vi "test-trapezoid-profile-top-speed.vi"() -> ()   [LabVIEW 2019]
uses:
  <vilib>/Rock Robotics/WPI/ThirdParty/JAS_Junk/TrajLib/TRAPEZOID_PROFILE_STATE.ctl
  <vilib>/Rock Robotics/WPI/ThirdParty/JAS_Junk/TrajLib/TRAPEZOID_PROFILE.ctl
  <vilib>/Rock Robotics/WPI/ThirdParty/JAS_Junk/TrajLib/TRAPEZOID_PROFILE_CONSTRAINT.ctl
  <vilib>/Rock Robotics/WPI/ThirdParty/JAS_Junk/TrajLib/TrapProfile_ShouldFlipAcceleration.vi
  <vilib>/Rock Robotics/WPI/ThirdParty/JAS_Junk/TrajLib/TrapProfile_Direct.vi
  <vilib>/Rock Robotics/WPI/ThirdParty/JAS_Junk/TrajLib/Trajectory_Library.lvlib
panel:
  out "State 2":T1 {"Velocity" format="%16_6e"; "Position" format="%16_6e"}
  out "Waveform Chart 2":T2(graph)
  out "TRAPEZOID_PROFILE 2":T3 {"Goal"."Velocity" format="%16_6e"; "Goal"."Position" format="%16_6e"; "Initial"."Velocity" format="%16_6e"; "Initial"."Position" format="%16_6e"; "Constraints"."MaxAcceleration" format="%16_6e"; "Constraints"."MaxVelocity" format="%16_6e"; "EndDecel" format="%16_6e"; "EndFullSpeed" format="%16_6e"; "EndAccel" format="%16_6e"}
  out "TRAPEZOID_PROFILE":T3 {"Goal"."Velocity" format="%16_6e"; "Goal"."Position" format="%16_6e"; "Initial"."Velocity" format="%16_6e"; "Initial"."Position" format="%16_6e"; "Constraints"."MaxAcceleration" format="%16_6e"; "Constraints"."MaxVelocity" format="%16_6e"; "EndDecel" format="%16_6e"; "EndFullSpeed" format="%16_6e"; "EndAccel" format="%16_6e"}
  out "State":T1 {"Velocity" format="%16_6e"; "Position" format="%16_6e"}
  out "Waveform Chart":T2(graph)
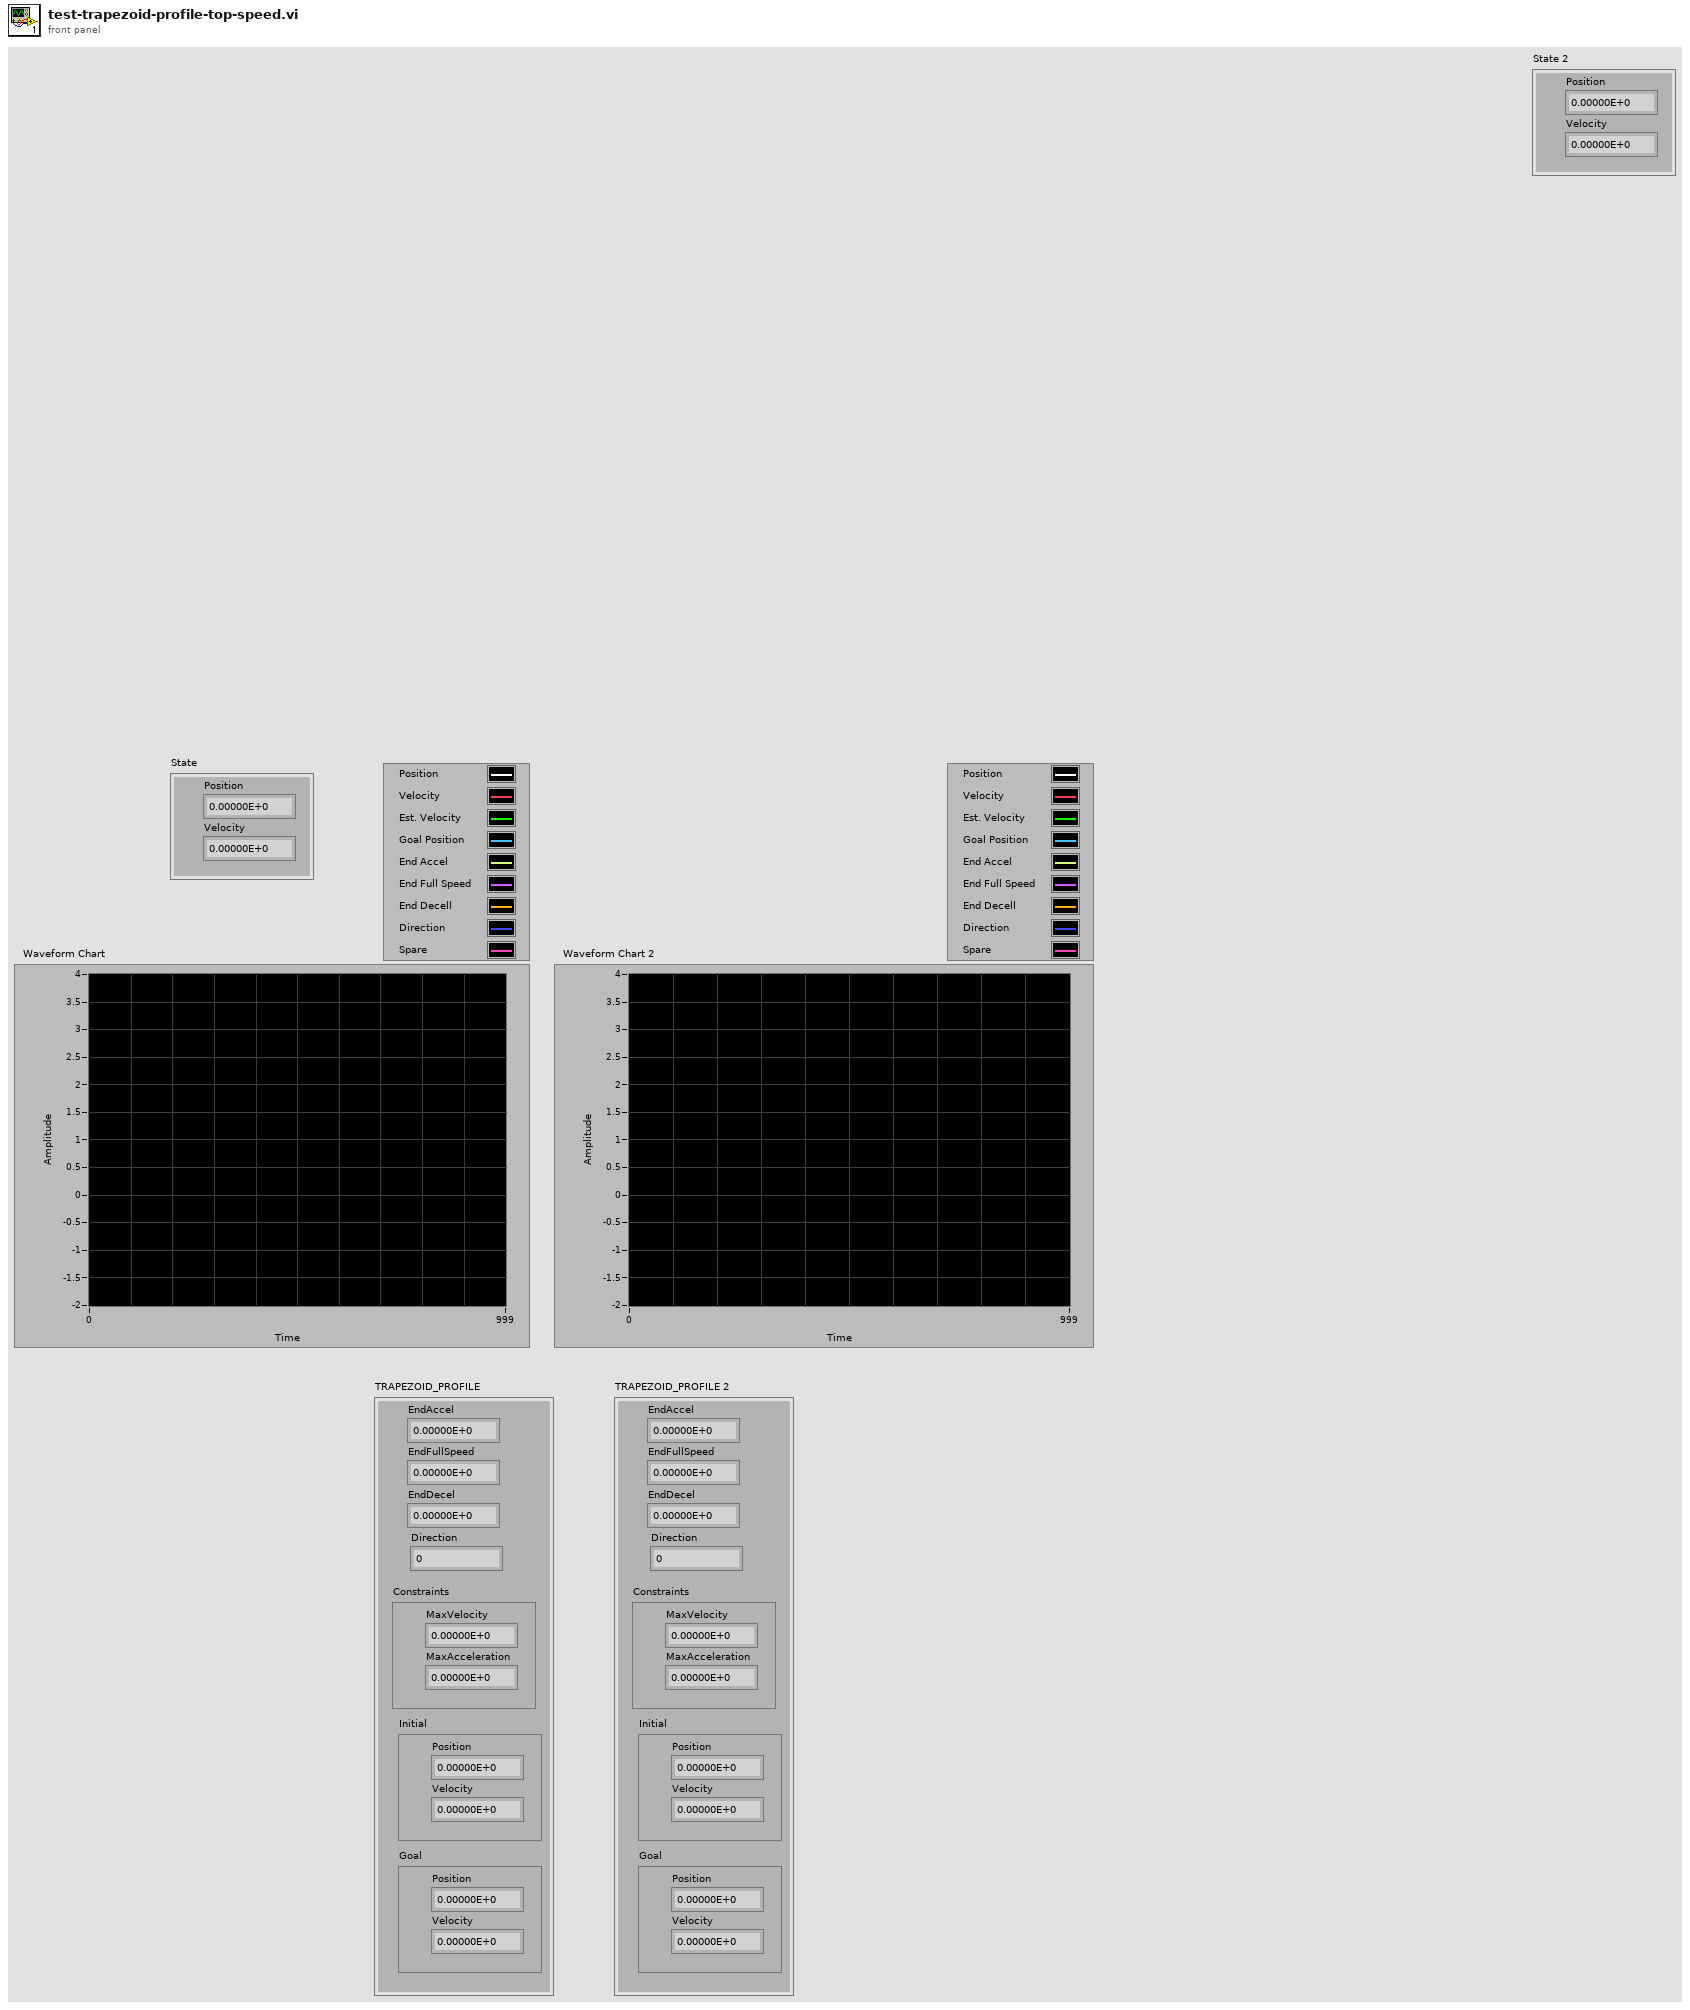
[diagram p1: front panel]
types:
  T1 = typedef "Trajectory_Library.lvlib/TRAPEZOID_PROFILE_STATE.ctl" = cluster{"Position":dbl, "Velocity":dbl}
  T2 = cluster{"Position":dbl, "Velocity":dbl, dbl, "Position":dbl, "EndAccel":dbl, "EndFullSpeed":dbl, "EndDecel":dbl, "Direction":i32, "Position":dbl}
  T3 = typedef "Trajectory_Library.lvlib/TRAPEZOID_PROFILE.ctl" = cluster{"EndAccel":dbl, "EndFullSpeed":dbl, "EndDecel":dbl, "Direction":i32, "Constraints":T4, "Initial":T1, "Goal":T1}
  T4 = typedef "Trajectory_Library.lvlib/TRAPEZOID_PROFILE_CONSTRAINT.ctl" = cluster{"MaxVelocity":dbl, "MaxAcceleration":dbl}
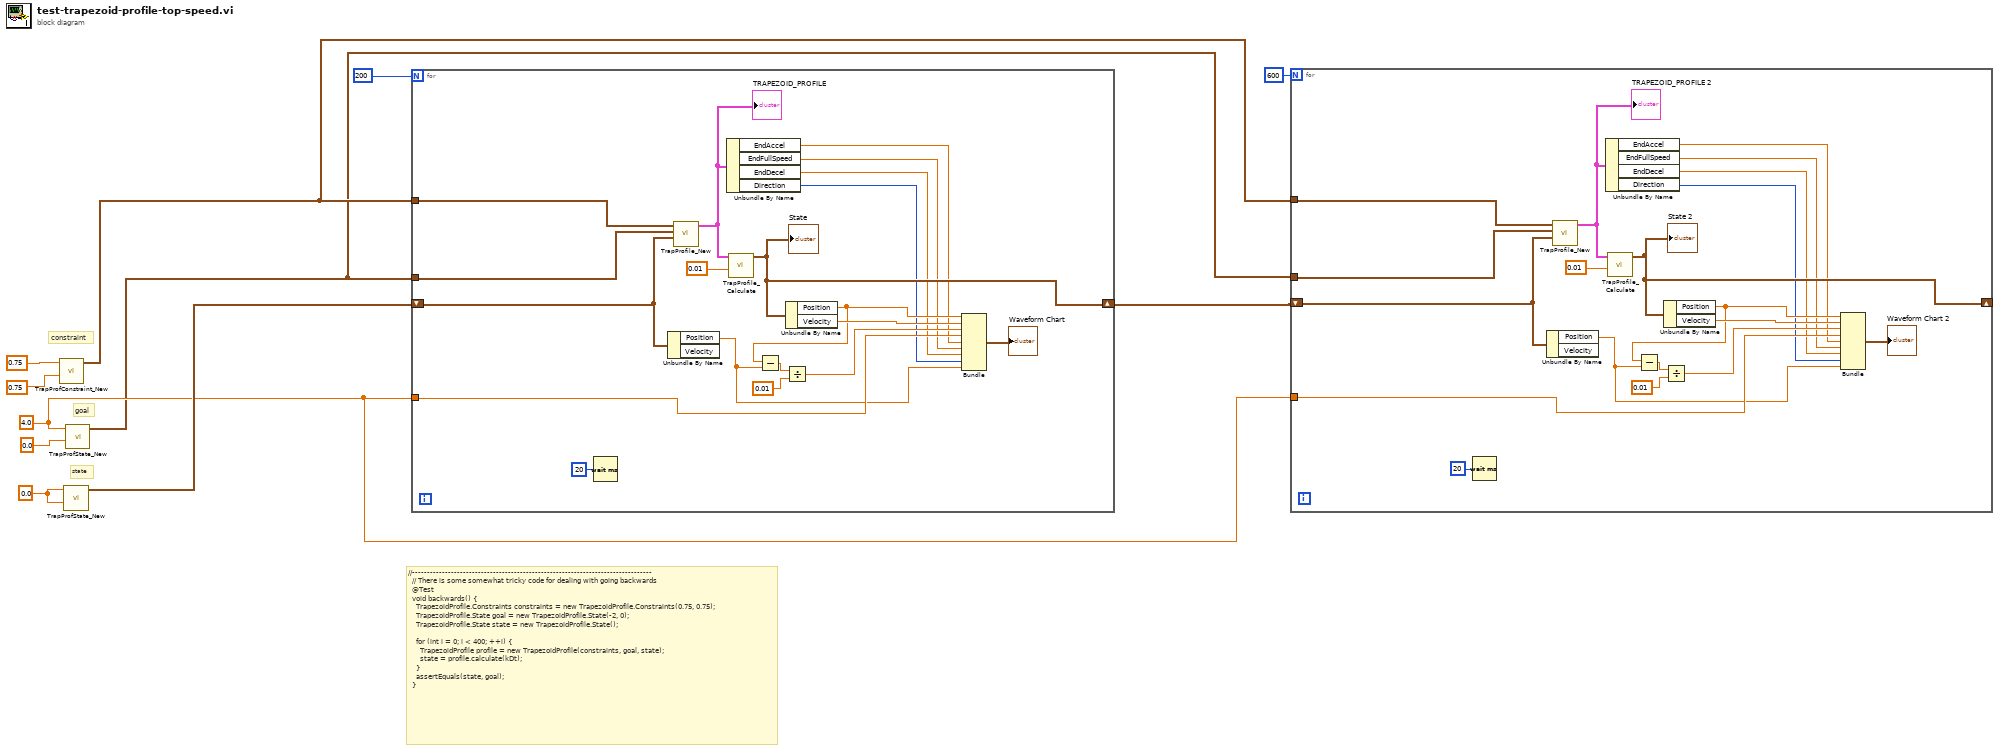
[diagram p0: block diagram]
diagram:
  w7 = 0.0 ("Position")
  w2 = 4.0 ("Position")
  # "state"
  # "//--------------------------------------------------------------------------------\n  // There is some somewhat tricky code for dealing with going backwards\n  @Test\n  void backwards() {\n    TrapezoidProfile.Constraints constraints = new TrapezoidProfile.Constraints(0.75, 0.75);\n    TrapezoidProfile.State goal = new TrapezoidProfile.State(-2, 0);\n    TrapezoidProfile.State state = new TrapezoidProfile.State();\n\n    for (int i = 0; i < 400; ++i) {\n      TrapezoidProfile profile = new TrapezoidProfile(constraints, goal, state);\n      state = profile.calculate(kDt);\n    }\n    assertEquals(state, goal);\n  }"
  # "goal"
  # "constraint"
  n1 = call <vilib>:"TrapProfConstraint_New.vi"("Max Accel"=0.75, "Max Speed (M/S)"=0.75) -> ("TRAPEZOID_PROFILE_CONSTRAINT"=w3:T4)  [unwired: 9 in]
  n2 = call <vilib>:"TrapProfState_New.vi"("Velocity"=w7, "Position"=w7) -> ("TRAPEZOID_PROFILE_STATE"=w6:T1)  [unwired: 9 in]
  n3 = call <vilib>:"TrapProfState_New.vi"("Velocity"=0.0, "Position"=w2) -> ("TRAPEZOID_PROFILE_STATE"=w1:T1)  [unwired: 9 in]
  n4 = for {
    N: 200 -> [_]
    shift-right: [w20] -> w4
    shift-left: w6 -> [w25]
    tunnel: w1 -> [w27]
    tunnel: w2 -> [w19]
    tunnel: w3 -> [w12]
    n5 = Wait (ms)(milliseconds to wait=u32 20) -> ()  [unwired: 1 out]
    n6 = Unbundle By Name(w25) -> ("Position"=w13:dbl)  [unwired: 1 out]
    n7 = call <vilib>:"TrapProfile_New.vi"("Initial"=w25, "Goal"=w27, "Constraints"=w12) -> ("TRAPEZOID_PROFILE"=w18:T3)  [unwired: 8 in]
    "TRAPEZOID_PROFILE" <- w18
    n8 = Unbundle By Name(w18) -> ("EndAccel"=w17:dbl, "EndFullSpeed"=w16:dbl, "EndDecel"=w15:dbl, "Direction"=w14:i32)
    n9 = call <vilib>:"TrapProfile_Calculate.vi"("Time"=0.01, "TRAPEZOID_PROFILE"=w18) -> ("State"=w20:T1)  [unwired: 9 in]
    "State" <- w20
    n10 = Unbundle By Name(w20) -> ("Position"=w24:dbl, "Velocity"=w28:dbl)
    n11 = Subtract(x=w24, y=w13) -> (x-y=w23:dbl)
    n12 = Divide(x=w23, y=0.01) -> (x/y=w21:dbl)
    n13 = Bundle("Position"=w24, "Velocity"=w28, w21, "Position"=w19, "EndAccel"=w17, "EndFullSpeed"=w16, "EndDecel"=w15, "Direction"=w14, "Position"=w13) -> (→"Waveform Chart":T2)  [unwired: 1 in]
  }
  n14 = for {
    N: 600 -> [_]
    shift-right: [w39] -> _
    shift-left: w4 -> [w44]
    tunnel: w1 -> [w46]
    tunnel: w2 -> [w38]
    tunnel: w3 -> [w31]
    n15 = Wait (ms)(milliseconds to wait=u32 20) -> ()  [unwired: 1 out]
    n16 = Unbundle By Name(w44) -> ("Position"=w32:dbl)  [unwired: 1 out]
    n17 = call <vilib>:"TrapProfile_New.vi"("Initial"=w44, "Goal"=w46, "Constraints"=w31) -> ("TRAPEZOID_PROFILE"=w37:T3)  [unwired: 8 in]
    "TRAPEZOID_PROFILE 2" <- w37
    n18 = Unbundle By Name(w37) -> ("EndAccel"=w36:dbl, "EndFullSpeed"=w35:dbl, "EndDecel"=w34:dbl, "Direction"=w33:i32)
    n19 = call <vilib>:"TrapProfile_Calculate.vi"("Time"=0.01, "TRAPEZOID_PROFILE"=w37) -> ("State"=w39:T1)  [unwired: 9 in]
    "State 2" <- w39
    n20 = Unbundle By Name(w39) -> ("Position"=w43:dbl, "Velocity"=w47:dbl)
    n21 = Subtract(x=w43, y=w32) -> (x-y=w42:dbl)
    n22 = Divide(x=w42, y=0.01) -> (x/y=w40:dbl)
    n23 = Bundle("Position"=w43, "Velocity"=w47, w40, "Position"=w38, "EndAccel"=w36, "EndFullSpeed"=w35, "EndDecel"=w34, "Direction"=w33, "Position"=w32) -> (→"Waveform Chart 2":T2)  [unwired: 1 in]
  }
